vi "CSM - Run Script with Local Variable Support.vi"(0 "CSM Scripts":string, 1 "Current Module (\"\" to Generate an ID)":string, 7 "Continue If Error? (F)":bool, 9 "Wait (5000ms)":i32=5000, 11 "error in (no error)":errorcluster, 12 "Response Timeout (-2 Using Global Settings)":i32=-2) -> (4 "Response":string[](array[string]), 10 "Scripts Left":string, 15 "error out":errorcluster)   [LabVIEW 2020]
doc: "Executes multiple CSM commands in a single batch, supporting synchronous messages, asynchronous messages, and registrations.\n\n\n> [!NOTE] <b>CSM Message Target Module Description</b>\n>\n> In Normal Mode, the target module for a CSM message is the specified module name.\n> System-level modules start with a `.` in their name. The target module for a CSM message includes the `.` in the name. For example, if the requested module name is `.System`, the target module for the CSM message is `.System`.\n> In Worker Mode, the target module for a CSM message can only be the overall module name, not the node name. For example, if the requested module name is `Worker#`, the target module for the CSM message is `Worker`.\n> In Chain of Responsibility Mode, the target module for a CSM message can only be the overall module name, not the node name. For example, if the requested module name is `Chain$1`, the target module for the CSM message is `Chain`.\n\n\n-- <b>Controls</b> --\n- <b>Current Module (\"\" to Generate an ID)</b>: Name of the current module. If empty, a temporary ID is generated for debugging purposes to identify the location.\n- <b>CSM Scripts</b>: CSM commands to execute.\n- <b>Continue If Error? (F)</b>: Whether to continue execution if an error occurs. The default is FALSE, which specifies to not continue.\n- <b>Wait (5000 ms)</b>: Timeout duration for waiting module to be alive. The default is 5000 ms.\n- <b>Response Timeout (-2 Using Global Settings)</b>: Timeout for synchronous calls. The default is -2, which uses the global setting. You can set the global timeout using the CSM - Set TMO of Sync-Reply VI.\n\n-- <b>Indicators</b> --\n- <b>Response</b>: Returned results from executing the script. Only synchronous messages carry returns. The corresponding column for other commands will be an empty string.\n- <b>Scripts Left</b>: Remaining unexecuted scripts."
uses:
  <userlib>/_NEVSTOP/Communicable State Machine(CSM)/AdvanceAPI/CSM - Broadcast Message Type.ctl
  <userlib>/_NEVSTOP/Communicable State Machine(CSM)/Communicable State Machine.lvlib
  <userlib>/_NEVSTOP/Communicable State Machine(CSM)/_Shared/CSM Shared.lvlib
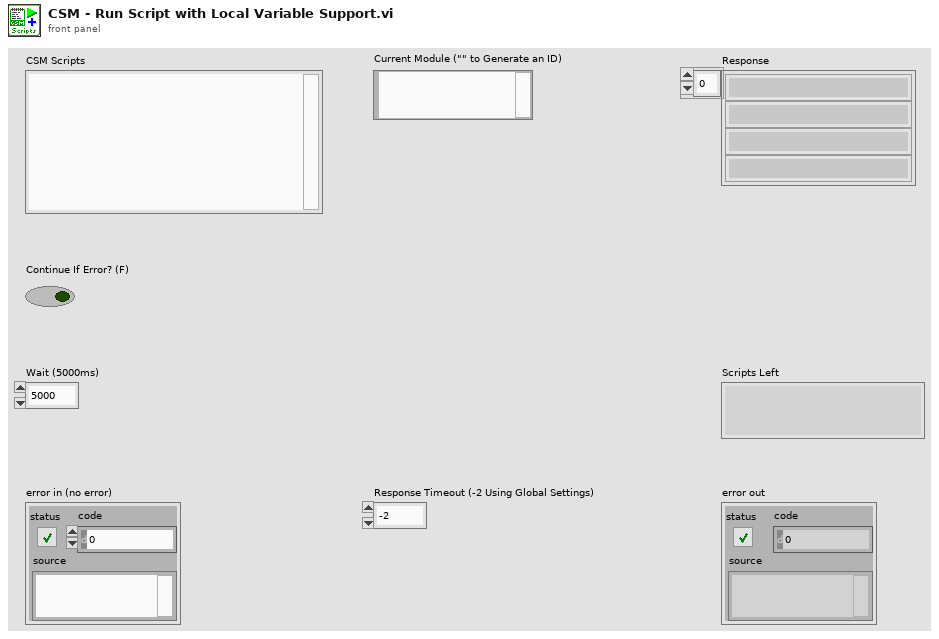
[diagram p1: front panel]
types:
  T1 = typedef "Communicable State Machine.lvlib/CSM - Broadcast Message Type.ctl" = enum16{"<Null>", "Status", "Interrupt"}
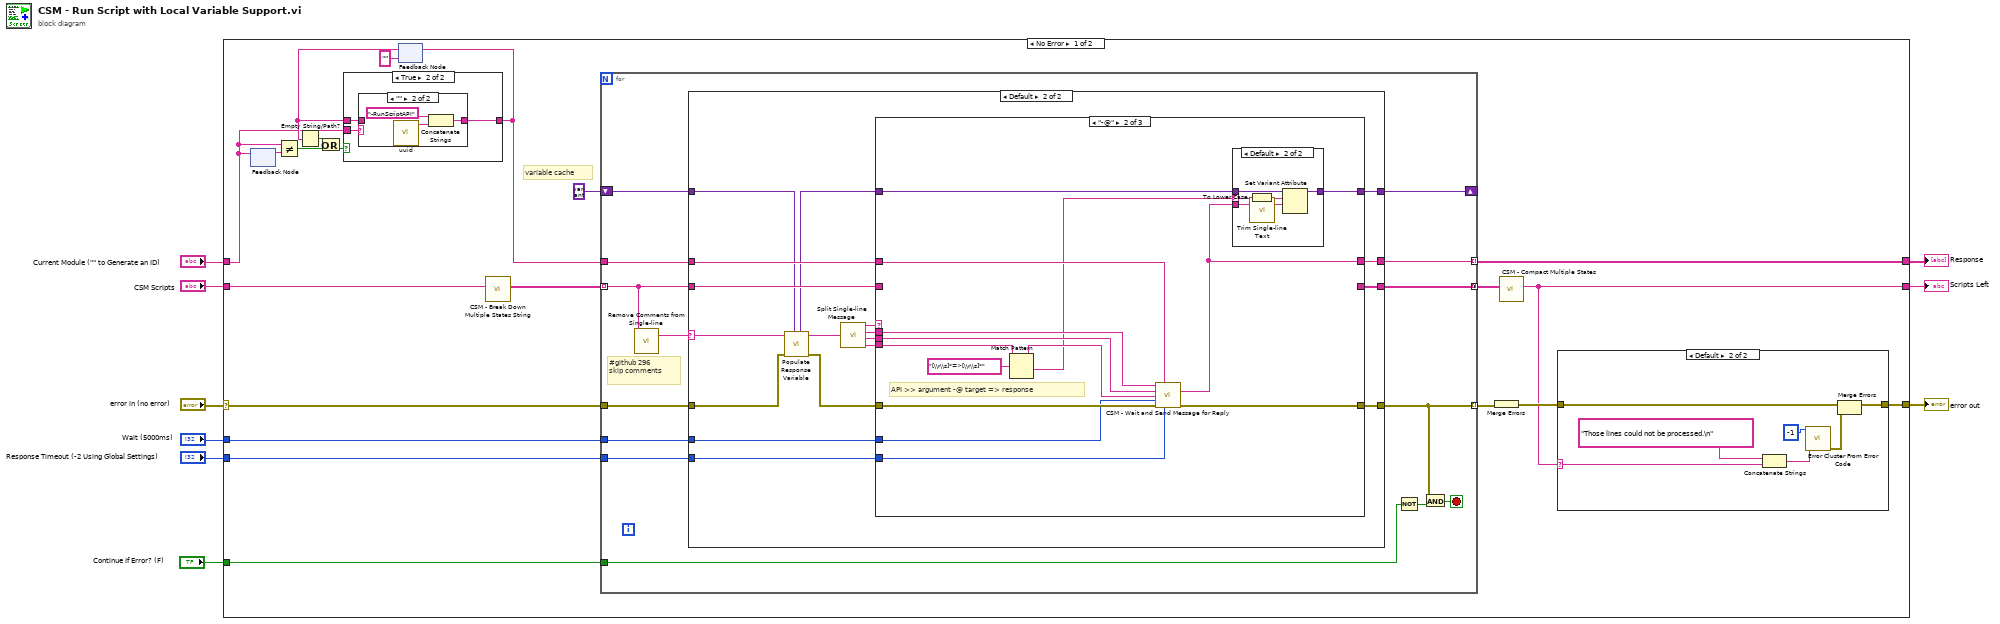
[diagram p0: block diagram]
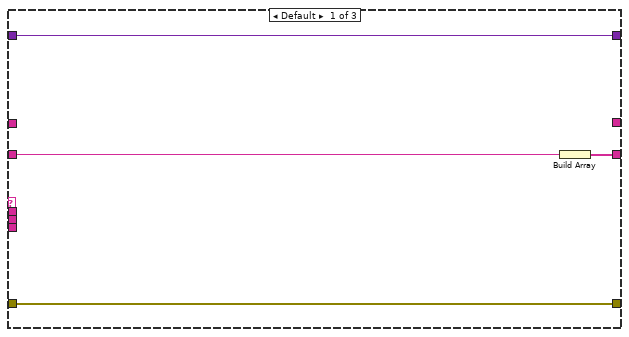
[diagram p6: hidden frame]
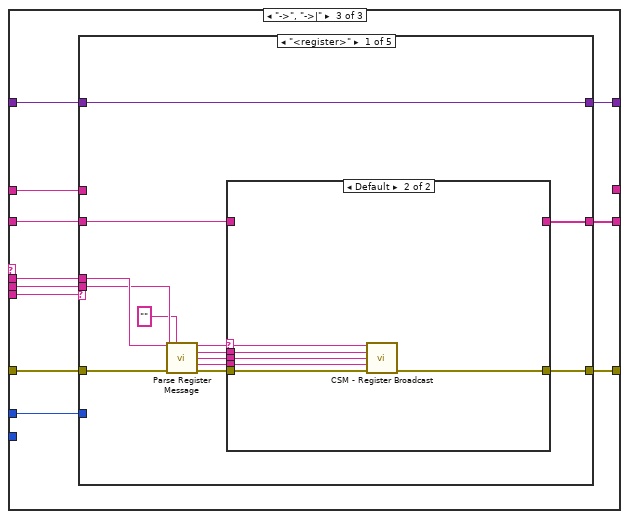
[diagram p8: hidden frame]
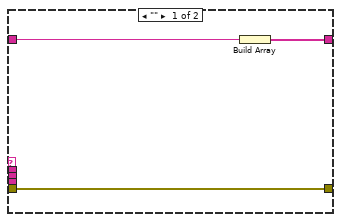
[diagram p9: hidden frame]
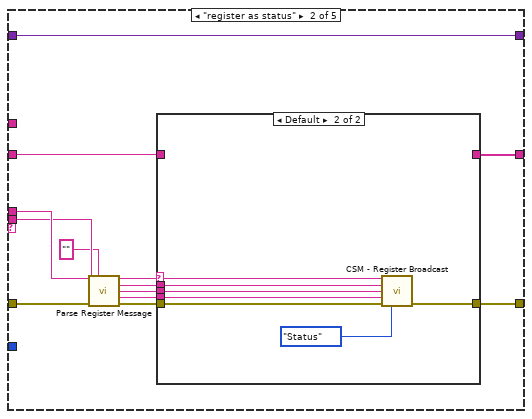
[diagram p10: hidden frame]
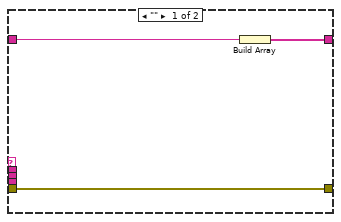
[diagram p11: hidden frame]
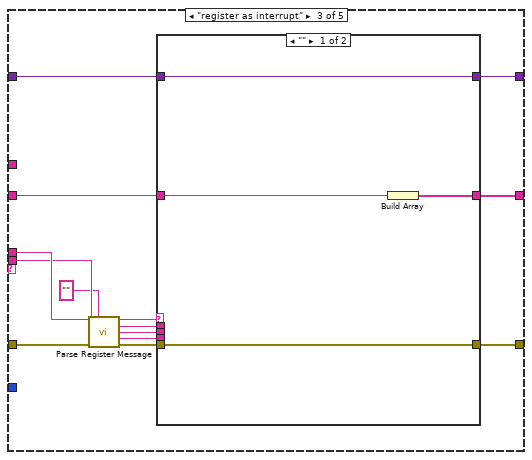
[diagram p12: hidden frame]
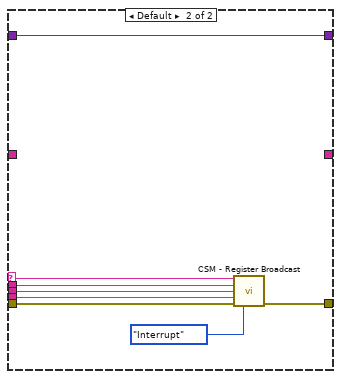
[diagram p13: hidden frame]
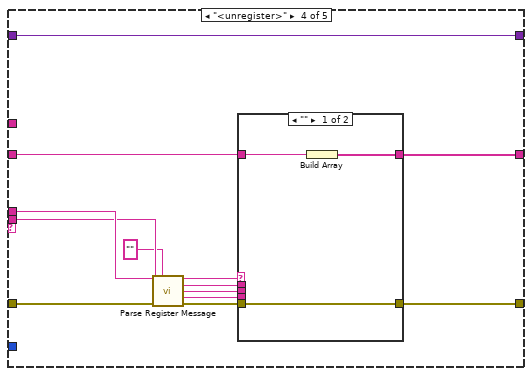
[diagram p14: hidden frame]
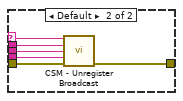
[diagram p15: hidden frame]
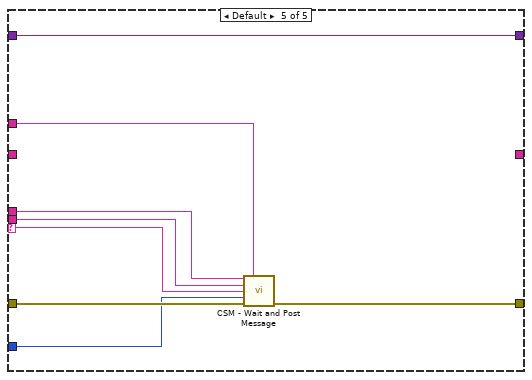
[diagram p16: hidden frame]
diagram:
  n1 = case shown="No Error" "error in (no error)" {
    selector: "error in (no error)" -> [w28 w214]
    tunnel: "CSM Scripts" -> [w27 _]
    tunnel: [w24 _] -> w7
    tunnel: [w23 w214] -> w6
    tunnel: "Current Module (\"\" to Generate an ID)" -> [w12 _]
    tunnel: "Response Timeout (-2 Using Global Settings)" -> [w22 _]
    tunnel: "Wait (5000ms)" -> [w21 _]
    tunnel: "Continue If Error? (F)" -> [w20 _]
    tunnel: [w19 _] -> w1
    frame No Error {
      # "variable cache"
      n2 = feedback #1() -> (w18:string)  [unwired: 1 in]
      n3 = feedback-in #1(w12) -> ()
      n4 = Not Equal?(x=w12, y=w18) -> (x != y?=w17:bool)
      n5 = feedback #2("") -> (w14:string)
      n6 = Empty String/Path?(string/path=w14) -> (empty?=w13:bool)
      n7 = Or(x=w13, y=w17) -> (x .or. y?=w15:bool)
      n8 = case shown="True" w15 {
        tunnel: w14 -> [w31 w34]
        tunnel: w12 -> [_ w33]
        tunnel: [w31 w32] -> w11
        frame False {
        }
        frame True {
          n9 = case shown="\"\"" w33 {
            selector: w33 -> [w35 _]
            tunnel: [w35 w36] -> w32
            tunnel: w34 -> [_ _]
            frame Default {
            }
            frame "" {
              n10 = call <userlib>:"uuid.vi"() -> ("UUID"=w37:string)  [unwired: 11 in]
              n11 = Concatenate Strings("-RunScriptAPI" ("Name (\"\" to Use UUID)"), w37) -> (w36:string)
            }
          }
        }
      }
      n12 = feedback-in #2(w11) -> ()
      n13 = call <userlib>:"CSM - Break Down Multiple States String.vi"("States"=w27) -> ("Multiple States"=w26:string[])  [unwired: 10 in]
      n14 = for {
        tunnel: w26 -> [w57] mode=indexing
        tunnel: w28 -> [w60]
        tunnel: [w52] -> w29 mode=indexing
        tunnel: [w58] -> w25 mode=concatenating
        tunnel: w11 -> [w56]
        tunnel: w22 -> [w55]
        tunnel: w21 -> [w54]
        tunnel: w20 -> [w51]
        tunnel: [w49] -> w19 mode=indexing
        shift-right: [w47] -> _
        shift-left: variant -> [w48]
        stop <- w53 stop-if-true
        # "#github 296\nskip comments"
        n15 = call <userlib>:"Remove Comments from Single-line.vi"("single-line text"=w57) -> ("single-line text without comments"=w59:string)  [unwired: 2 in]
        n16 = case shown="Default" w59 {
          selector: w59 -> [_ w66]
          tunnel: [w62 w80] -> w52
          tunnel: w60 -> [w62 w64]
          tunnel: [_ w75] -> w58
          tunnel: w57 -> [_ w74]
          tunnel: w56 -> [_ w73]
          tunnel: w55 -> [_ w72]
          tunnel: w54 -> [_ w71]
          tunnel: [_ w70] -> w49
          tunnel: w48 -> [w61 w68]
          tunnel: [w61 w69] -> w47
          frame "" {
          }
          frame Default {
            n17 = call "Populate Response Variable.vi"("Variant"=w68, "Error in"=w64, "String might with variables"=w66) -> ("Error out"=w63:errorcluster, "String out"=w65:string, "Variant Out"=w67:variant)  [unwired: 4 in]
            n18 = call <userlib>:"Split Single-line Message.vi"("single-line text"=w65) -> ("operator"=w79:string, "state"=w76:string, "args"=w77:string, "source/target"=w78:string)  [unwired: 6 in]
            n19 = case shown="\"-@\"" w79 {
              tunnel: w78 -> [_ w91 w116]
              tunnel: w77 -> [_ w98 w115]
              tunnel: w76 -> [_ w97 w114]
              tunnel: w63 -> [w84 w96 w113]
              tunnel: [w84 w95 w112] -> w80
              tunnel: [w83 _ w111] -> w75
              tunnel: w74 -> [w82 _ w110]
              tunnel: w73 -> [_ w94 w109]
              tunnel: w72 -> [_ w93 _]
              tunnel: w71 -> [_ w92 w108]
              tunnel: [_ w85 _] -> w70
              tunnel: [w81 w87 w107] -> w69
              tunnel: w67 -> [w81 w88 w106]
              frame Default {
                n20 = Build Array(w82) -> (w83:string[])
              }
              frame "-@" {
                # "API >> argument -@ target => response"
                n21 = Match Pattern(string=w91, regular expression="[\\r\\s]*=>[\\r\\s]*") -> (before substring=w89:string, after substring=w86:string)  [unwired: 1 in, 2 out]
                n22 = call <userlib>:"CSM - Wait and Send Message for Reply.vi"("State"=w97, "Current Module (\"\" to Generate an ID)"=w94, "Arguments (\"\")"=w98, "Target Module"=w89, "Wait (5000ms)"=w92, "Error In (No Error)"=w96, "Response Timeout (-2 Using Global Settings)"=w93) -> ("Response"=w85:string, "error out"=w95:errorcluster)  [unwired: 5 in, 2 out]
                n23 = case shown="Default" w86 {
                  selector: w86 -> [_ w103]
                  tunnel: w88 -> [w99 w105]
                  tunnel: [w99 w104] -> w87
                  tunnel: w85 -> [_ w102]
                  frame "" {
                  }
                  frame Default {
                    n24 = To Lower Case(string=w103) -> (all lower case string=w100:string)
                    n25 = call <userlib>:"Trim Single-line Text.vi"("single-line text"=w102) -> ("trimed text"=w101:string)  [unwired: 2 in]
                    n26 = Set Variant Attribute(Variant=w105, name=w100, value=w101) -> (Variant out=w104:variant)  [unwired: 1 in, 2 out]
                  }
                }
              }
              frame "->", "->|" {
                n27 = case shown="\"<register>\"" w116 {
                  selector: w116 -> [_ _ _ _ w213]
                  tunnel: w115 -> [w123 w144 w167 w191 w212]
                  tunnel: w114 -> [w124 w145 w168 w192 w211]
                  tunnel: w113 -> [w122 w143 w166 w190 w210]
                  tunnel: [w121 w142 w165 w189 w209] -> w112
                  tunnel: [w119 w140 w163 w187 _] -> w111
                  tunnel: w110 -> [w118 w139 w162 w186 _]
                  tunnel: w109 -> [_ _ _ _ w208]
                  tunnel: w108 -> [_ _ _ _ w207]
                  tunnel: [w117 w138 w161 w185 w206] -> w107
                  tunnel: w106 -> [w117 w138 w160 w185 w206]
                  frame "<register>" {
                    n28 = call <userlib>:"Parse Register Message.vi"("State"=w124, "Module Name"="", "Args"=w123) -> ("Target"=w128:string, "Source"=w127:string, "Status"=w126:string, "Api"=w125:string)  [unwired: 8 in, 1 out]
                    n29 = case shown="Default" w128 {
                      selector: w128 -> [_ w137]
                      tunnel: w127 -> [_ w136]
                      tunnel: w126 -> [_ w135]
                      tunnel: w125 -> [_ w134]
                      tunnel: w122 -> [w131 w133]
                      tunnel: [w131 w132] -> w121
                      tunnel: [w129 _] -> w119
                      tunnel: w118 -> [w130 _]
                      frame "" {
                        n30 = Build Array(w130) -> (w129:string[])
                      }
                      frame Default {
                        n31 = call <userlib>:"CSM - Register Broadcast.vi"("CSM Name(Empty for Broadcast Event)"=w137, "Source CSM Name (* as Default)"=w136, "Trigger"=w135, "API (If \"\", Same as Trigger)"=w134, "Error In"=w133) -> ("error out"=w132:errorcluster)  [unwired: 9 in, 1 out]
                      }
                    }
                  }
                  frame "register as status" {
                    n32 = call <userlib>:"Parse Register Message.vi"("State"=w145, "Module Name"="", "Args"=w144) -> ("Target"=w149:string, "Source"=w148:string, "Status"=w147:string, "Api"=w146:string)  [unwired: 8 in, 1 out]
                    n33 = case shown="Default" w149 {
                      selector: w149 -> [_ w159]
                      tunnel: w148 -> [_ w158]
                      tunnel: w147 -> [_ w157]
                      tunnel: w146 -> [_ w156]
                      tunnel: w143 -> [w152 w155]
                      tunnel: [w152 w154] -> w142
                      tunnel: [w150 _] -> w140
                      tunnel: w139 -> [w151 _]
                      frame "" {
                        n34 = Build Array(w151) -> (w150:string[])
                      }
                      frame Default {
                        n35 = call <userlib>:"CSM - Register Broadcast.vi"("CSM Name(Empty for Broadcast Event)"=w159, "Source CSM Name (* as Default)"=w158, "Trigger"=w157, "API (If \"\", Same as Trigger)"=w156, "Error In"=w155, "Priority (No Change)"=CSM_-_Broadcast_Message_Type."Status") -> ("error out"=w154:errorcluster)  [unwired: 8 in, 1 out]
                      }
                    }
                  }
                  frame "register as interrupt" {
                    n36 = call <userlib>:"Parse Register Message.vi"("State"=w168, "Module Name"="", "Args"=w167) -> ("Target"=w172:string, "Source"=w171:string, "Status"=w170:string, "Api"=w169:string)  [unwired: 8 in, 1 out]
                    n37 = case shown="\"\"" w172 {
                      selector: w172 -> [_ w184]
                      tunnel: w171 -> [_ w183]
                      tunnel: w170 -> [_ w182]
                      tunnel: w169 -> [_ w181]
                      tunnel: w166 -> [w176 w180]
                      tunnel: [w176 w179] -> w165
                      tunnel: [w174 _] -> w163
                      tunnel: w162 -> [w175 _]
                      tunnel: [w173 w177] -> w161
                      tunnel: w160 -> [w173 w177]
                      frame "" {
                        n38 = Build Array(w175) -> (w174:string[])
                      }
                      frame Default {
                        n39 = call <userlib>:"CSM - Register Broadcast.vi"("CSM Name(Empty for Broadcast Event)"=w184, "Source CSM Name (* as Default)"=w183, "Trigger"=w182, "API (If \"\", Same as Trigger)"=w181, "Error In"=w180, "Priority (No Change)"=CSM_-_Broadcast_Message_Type."Interrupt") -> ("error out"=w179:errorcluster)  [unwired: 8 in, 1 out]
                      }
                    }
                  }
                  frame "<unregister>" {
                    n40 = call <userlib>:"Parse Register Message.vi"("State"=w192, "Module Name"="", "Args"=w191) -> ("Target"=w196:string, "Source"=w195:string, "Status"=w194:string, "Api"=w193:string)  [unwired: 8 in, 1 out]
                    n41 = case shown="\"\"" w196 {
                      selector: w196 -> [_ w205]
                      tunnel: w195 -> [_ w204]
                      tunnel: w194 -> [_ w203]
                      tunnel: w193 -> [_ w202]
                      tunnel: w190 -> [w199 w201]
                      tunnel: [w199 w200] -> w189
                      tunnel: [w197 _] -> w187
                      tunnel: w186 -> [w198 _]
                      frame "" {
                        n42 = Build Array(w198) -> (w197:string[])
                      }
                      frame Default {
                        n43 = call <userlib>:"CSM - Unregister Broadcast.vi"("CSM Name(Empty for Broadcast Event)"=w205, "Source CSM Name (* as Default)"=w204, "Trigger"=w203, "API (\"*\" as Default)"=w202, "Error In"=w201) -> ("error out"=w200:errorcluster)  [unwired: 9 in, 1 out]
                      }
                    }
                  }
                  frame Default {
                    n44 = call <userlib>:"CSM - Wait and Post Message.vi"("State"=w211, "Current Module (\"\" to Generate an ID)"=w208, "Arguments (\"\")"=w212, "Target Module"=w213, "Wait (5000ms)"=w207, "Error In (No Error)"=w210) -> ("error out"=w209:errorcluster)  [unwired: 8 in, 1 out]
                  }
                }
              }
            }
          }
        }
        n45 = Not(x=w51) -> (.not. x?=w50:bool)
        n46 = And(x=w52, y=w50) -> (x .and. y?=w53:bool)
      }
      n47 = Merge Errors(w29) -> (w30:errorcluster)
      n48 = call <userlib>:"CSM - Compact Multiple States.vi"("Multiple States"=w25) -> ("States"=w24:string)  [unwired: 9 in]
      n49 = case shown="Default" w24 {
        selector: w24 -> [_ w42]
        tunnel: w30 -> [w39 w46]
        tunnel: [w39 w41] -> w23
        frame "" {
        }
        frame Default {
          n50 = Concatenate Strings("Those lines could not be processed.\n" ("String to Prepend to source (\"\")"), w42) -> (w43:string)
          n51 = call <vilib>:"Error Cluster From Error Code.vi"("error message (\"\")"=w43, "error code (0)"=-1 ("code")) -> ("error out"=w40:errorcluster)  [unwired: 7 in]
          n52 = Merge Errors(w46, w40) -> (w41:errorcluster)
        }
      }
    }
    frame Error {
    }
  }
  "error out" <- w6
  "Scripts Left" <- w7
  "Response" <- w1
